vi "test_Fix path.vi"(8 "error in (no error)":errorcluster, 11 "TestCase in":refnum<class "[Test Case] Fix path.lvclass">) -> (0 "error out":errorcluster, 3 "TestCase out":refnum<class "[Test Case] Fix path.lvclass">)   [LabVIEW 2015, in "Tests.lvlib" / "[Test Case] Fix path.lvclass"]
uses:
  [Test Case] Fix path.lvclass
  [Test Case] Fix path.lvclass/[Test Case] Fix path.ctl
  <vilib>/Utility/error.llb/Trim Whitespace.vi
  classes/File Transfer Behavior/File Transfer Behavior.lvclass
  <vilib>/addons/_JKI Toolkits/VI Tester/TestCase.llb/TestCase.lvclass
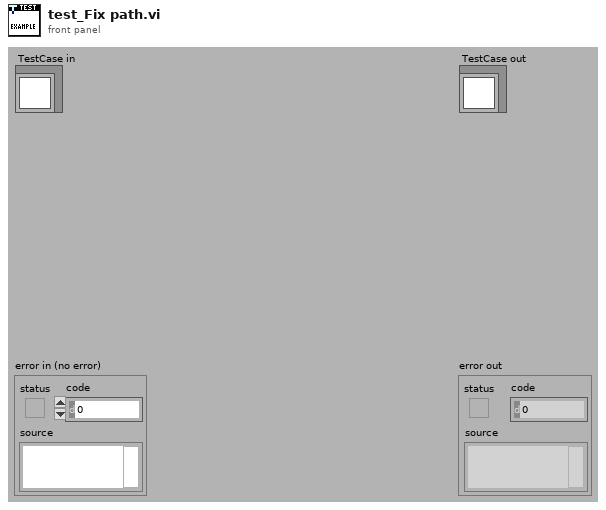
[diagram p1: front panel]
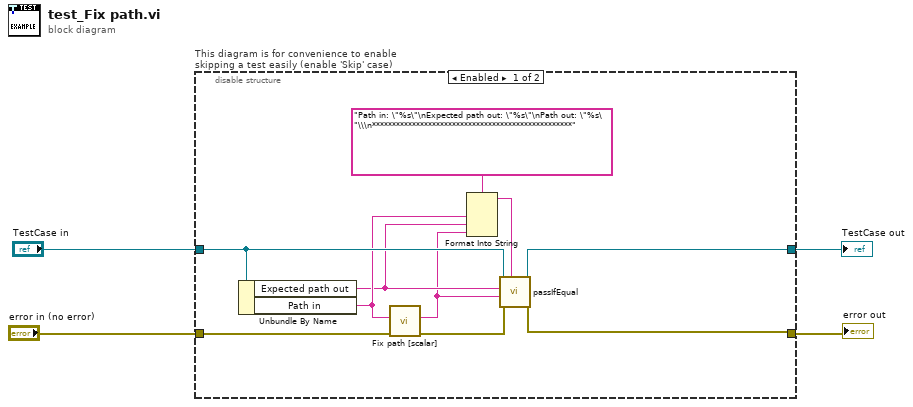
[diagram p0: block diagram]
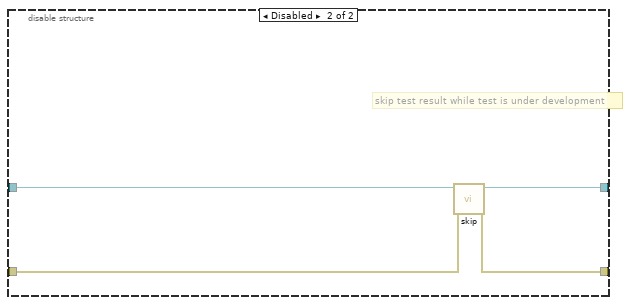
[diagram p2: hidden frame]
diagram:
  n1 = disable-structure "This diagram is for convenience to enable skipping a test easily (enable 'Skip' case)" shown="Enabled" {
    disable-tunnel: "TestCase in" -> [w10 w18]
    disable-tunnel: [w14 w16] -> w1
    disable-tunnel: [w13 w17] -> w3
    disable-tunnel: "error in (no error)" -> [w12 w15]
    frame Enabled {
      n2 = Unbundle By Name(w10) -> ("Expected path out"=w7:string, "Path in"=w8:string)
      n3 = call "Fix path [scalar].vi"("error in (no error)"=w12, "Path in"=w8) -> ("error out"=w11:errorcluster, "Path out"=w6:string)  [unwired: 7 in, 1 out]
      n4 = Format Into String(format string="Path in: \"%s\"\nExpected path out: \"%s\"\nPath out: \"%s\"\\\n**************************************************", w8, w7, w6) -> (resulting string=w5:string)  [unwired: 2 in, 1 out]
      n5 = call-dynamic "passIfEqual.vi"("custom report message (\"\")"=w5, "error in (no error)"=w11, "y"=w6, "x"=w7, "TestCase in"=w10) -> ("error out"=w13:errorcluster, "TestCase out"=w14:refnum<class "[Test Case] Fix path.lvclass">)  [unwired: 5 in]
    }
    frame Disabled {
      # "skip test result while test is under development"
      n6 = call <vilib>:"skip.vi"("error in (no error)"=w15, "TestCase in"=w18) -> ("error out"=w17:errorcluster, "TestCase out"=w16:refnum<class "[Test Case] Fix path.lvclass">)  [unwired: 8 in]
    }
  }
  "error out" <- w3
  "TestCase out" <- w1
